vi "Load Image From File.vi"(8 "错误输入（无错误）":errorcluster, 11 "Image Input Path":path) -> (0 "错误输出":errorcluster, 3 "FromFile":refnum<k24>)   [LabVIEW 2011, in "Image Converter.lvlib"]
uses:
  Image Converter.lvlib
  System.Drawing
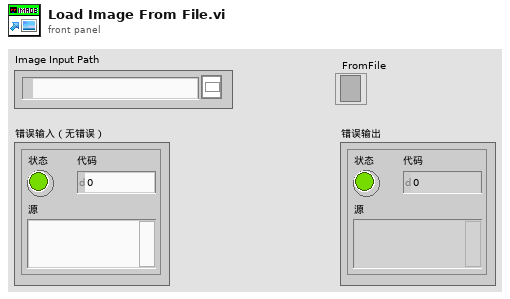
[diagram p1: front panel]
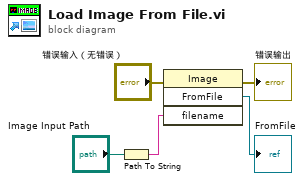
[diagram p0: block diagram]
diagram:
  n1 = Path To String(path="Image Input Path") -> (string=w1:string)
  n2 = invoke class="Image" method="FromFile"(error in="错误输入（无错误）", "filename"=w1) -> (error out=→"错误输出":errorcluster, "FromFile"=→"FromFile":refnum<k24>)  [unwired: 2 in, 2 out]
